vi "rtout_getTriggerConfig.vi"(0 "connection ID":refnum<k5>, 1 "axis":i32, 5 "error":errorcluster) -> (12 "polarity":i32, 14 "connection ID out":refnum<k5>, 15 "axis_out":i32, 16 "higher":i32, 17 "lower":i32, 18 "epsilon":i32, 19 "error out":errorcluster)   [LabVIEW 2016, in "amc_api.lvlib"]
doc: "Get the real time output trigger config"
uses:
  amc_api.lvlib
panel:
  out "jsonRespIn":string
  out "JSON-response":string="{\"jsonrpc\":\"2.0\",\"method\":\"\",\"params\":[5,1.245,true,\"name\"],\"id\":\"1\"}"
  out "JSON request":string
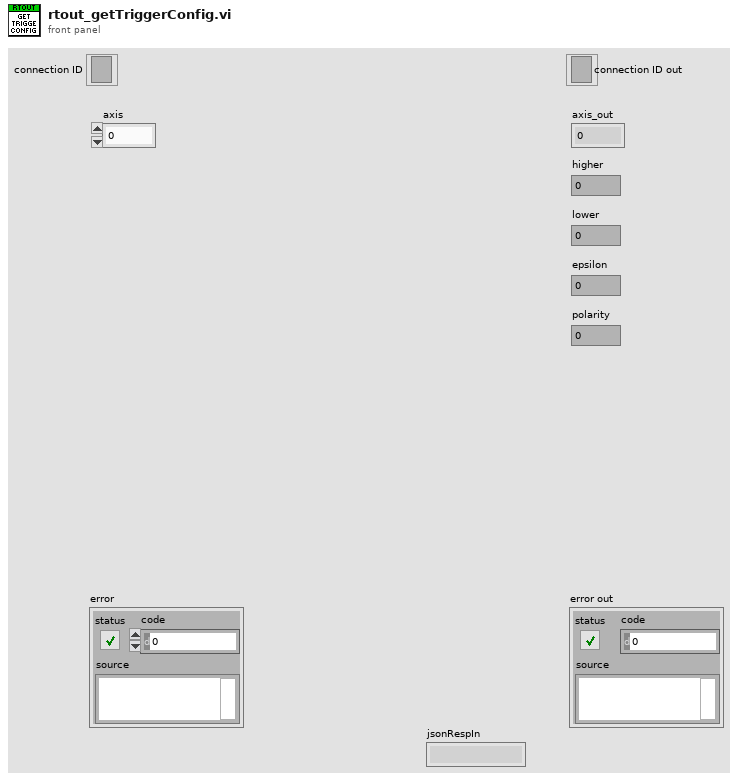
[diagram p1: front panel]
types:
  T1 = cluster{"jsonrpc":string, "method":string, "params":string[], "id":string, "api":i32, "pid":string}
  T2 = enum16{"Standard", "Buffered", "CRLF", "Immediate"}
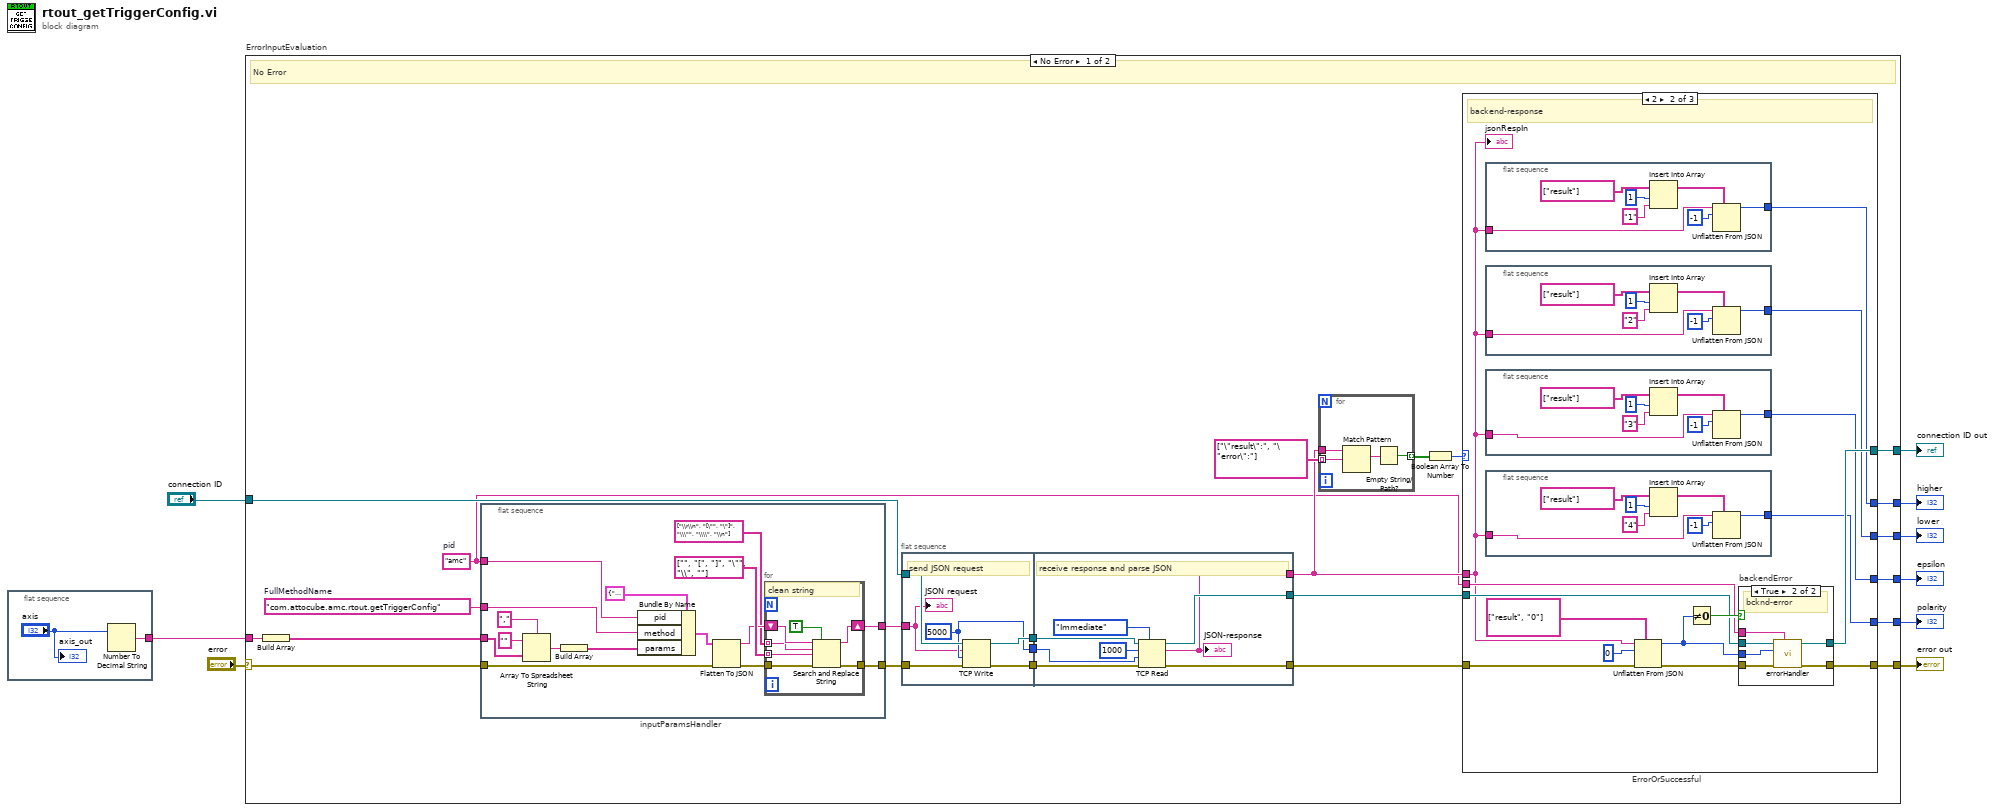
[diagram p0: block diagram]
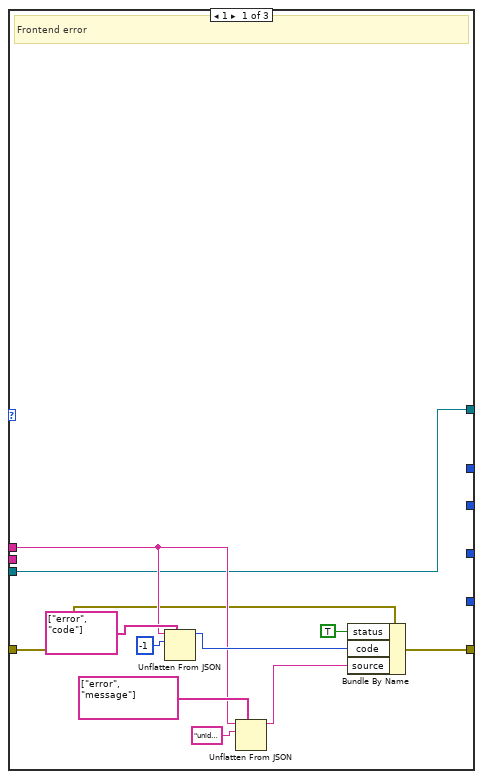
[diagram p2: hidden frame]
diagram:
  n1 = flat-sequence "in_axis" {
    tunnel: [w11] -> w5
    frame #0 {
      n2 = Number To Decimal String(number="axis") -> (decimal integer string=w11:string)  [unwired: 1 in]
      "axis_out" <- "axis"
    }
  }
  n3 = case "ErrorInputEvaluation" shown="No Error" "error" {
    selector: "error" -> [w27 w140]
    tunnel: "connection ID" -> [w31 w141]
    tunnel: [w18 w140] -> w8
    tunnel: [w19 w141] -> w7
    tunnel: w5 -> [w16 _]
    tunnel: [w15 _] -> w4
    tunnel: [w14 _] -> w3
    tunnel: [w13 _] -> w2
    tunnel: [w12 _] -> w1
    frame No Error {
      w17 = "amc"  # pid
      w28 = "com.attocube.amc.rtout.getTriggerConfig"  # FullMethodName
      # "No Error"
      n4 = Build Array ("ParametersArrayString")(w16) -> (w26:string[])
      n5 = flat-sequence "inputParamsHandler" {
        tunnel: [w104] -> w25
        tunnel: w26 -> [w110]
        tunnel: w27 -> [w109]
        tunnel: [w106] -> w24
        tunnel: w28 -> [w100]
        tunnel: w17 -> [w99]
        frame #0 {
          n6 = Array To Spreadsheet String(delimiter (Tab)=",", array=w110, 3:"" ("format string")) -> (spreadsheet string=w112:string)
          n7 = Build Array "Build Array"(w112) -> (w101:string[])
          n8 = Bundle By Name(cluster=T1 {"jsonrpc"="2.0", "method"="com.attocube.amc.res.setRESReadOutFreq", "params"=[], "id"="1", "api"=2, "pid"=""} ("Cluster"), "pid"=w99, "method"=w100, "params"=w101) -> (w111:T1)
          n9 = Flatten To JSON(anything=w111, error in (no error)=w109) -> (JSON string=w105:string, 11:w107:errorcluster)  [unwired: 1 in]
          n10 = for {
            tunnel: string[] ["\\r\\n", "[\"", "\"]", "\\\"", "\\\\", "\\n"] ("search string") -> [w118] mode=indexing
            tunnel: string[] ["", "[", "]", "\"", "\\", ""] ("replace string (\"\")") -> [w117] mode=indexing
            shift-right: [w120] -> w104
            shift-left: w105 -> [w119]
            tunnel: w107 -> [w116]
            tunnel: [w115] -> w106
            # "clean string"
            n11 = Search and Replace String(replace all?=TRUE ("replace all? (F)"), input string=w119, search string=w118, replace string=w117, error in=w116) -> (result string=w120:string, error out=w115:errorcluster)  [unwired: 3 in, 2 out]
          }
        }
      }
      n12 = flat-sequence {
        tunnel: w31 -> [w131]
        tunnel: [w129] -> w34
        tunnel: [w130] -> w33
        tunnel: w24 -> [w126]
        tunnel: [w128] -> w32
        tunnel: w25 -> [w127]
        tunnel: [w135] -> w23
        tunnel: w34 -> [w137]
        tunnel: w33 -> [w136]
        tunnel: [w133] -> w22
        tunnel: w32 -> [w134]
        tunnel: [w132] -> w21
        frame #0 {
          w128 = 5000 ("timeout ms (25000)")
          # "send JSON request"
          n13 = TCP Write(connection ID=w131, data in=w127, error in (no error)=w126, 9:w128) -> (connection ID out=w129:refnum<k5>, error out=w130:errorcluster)  [unwired: 1 out]
          "JSON request" <- w127
        }
        frame #1 {
          # "receive response and parse JSON"
          n14 = TCP Read(connection ID=w137, bytes to read=1000, error in (no error)=w136, 7:T2."Immediate" ("mode (standard)"), 9:w134) -> (connection ID out=w135:refnum<k5>, data out=w132:string, error out=w133:errorcluster)
          "JSON-response" <- w132
        }
      }
      n15 = for {
        tunnel: string[] ["\"result\":", "\"error\":"] ("path") -> [w124] mode=indexing
        tunnel: [w122] -> w29 mode=indexing
        tunnel: w21 -> [w125]
        n16 = Match Pattern(string=w125, regular expression=w124) -> (match substring=w123:string)  [unwired: 1 in, 3 out]
        n17 = Empty String/Path?(string/path=w123) -> (empty?=w122:bool)
      }
      n18 = Boolean Array To Number(Boolean array=w29) -> (number=w20:u32)
      n19 = case "ErrorOrSuccessful" shown="2" w20 {
        tunnel: w21 -> [w37 w52 _]
        tunnel: w23 -> [w35 w54 w98]
        tunnel: [w35 w53 w98] -> w19
        tunnel: [w38 w50 w97] -> w18
        tunnel: w22 -> [w36 w51 w97]
        tunnel: w17 -> [_ w55 _]
        tunnel: [_ w49 _] -> w15
        tunnel: [_ w48 _] -> w14
        tunnel: [_ w47 _] -> w13
        tunnel: [_ w46 _] -> w12
        frame 1 {
          # "Frontend error"
          n20 = Unflatten From JSON(path=string[] ["error", "code"], JSON string=w37, type and defaults=-1) -> (value=w44:i32)  [unwired: 4 in, 1 out]
          n21 = Unflatten From JSON(path=string[] ["error", "message"], JSON string=w37, type and defaults="unidentified error") -> (value=w45:string)  [unwired: 4 in, 1 out]
          n22 = Bundle By Name(cluster=w36, "status"=TRUE, "code"=w44, "source"=w45) -> (w38:errorcluster)
        }
        frame 2 {
          # "backend-response"
          n23 = flat-sequence "out_integer" {
            tunnel: w52 -> [w84]
            tunnel: [w82] -> w49
            frame #0 {
              n24 = Insert Into Array(array=string[] ["result"] ("path"), index=1, new element="1" ("idx")) -> (w86:string[])
              n25 = Unflatten From JSON(path=w86, JSON string=w84, type and defaults=-1 ("index")) -> (value=w82:i32)  [unwired: 4 in, 1 out]
            }
          }
          n26 = flat-sequence "out_integer" {
            tunnel: w52 -> [w77]
            tunnel: [w75] -> w48
            frame #0 {
              n27 = Insert Into Array(array=string[] ["result"] ("path"), index=1, new element="2" ("idx")) -> (w79:string[])
              n28 = Unflatten From JSON(path=w79, JSON string=w77, type and defaults=-1 ("index")) -> (value=w75:i32)  [unwired: 4 in, 1 out]
            }
          }
          n29 = flat-sequence "out_integer" {
            tunnel: w52 -> [w70]
            tunnel: [w68] -> w47
            frame #0 {
              n30 = Insert Into Array(array=string[] ["result"] ("path"), index=1, new element="3" ("idx")) -> (w72:string[])
              n31 = Unflatten From JSON(path=w72, JSON string=w70, type and defaults=-1 ("index")) -> (value=w68:i32)  [unwired: 4 in, 1 out]
            }
          }
          n32 = flat-sequence "out_integer" {
            tunnel: w52 -> [w63]
            tunnel: [w61] -> w46
            frame #0 {
              n33 = Insert Into Array(array=string[] ["result"] ("path"), index=1, new element="4" ("idx")) -> (w65:string[])
              n34 = Unflatten From JSON(path=w65, JSON string=w63, type and defaults=-1 ("index")) -> (value=w61:i32)  [unwired: 4 in, 1 out]
            }
          }
          n35 = Unflatten From JSON(path=string[] ["result", "0"], JSON string=w52, type and defaults=0, error in (no error)=w51) -> (value=w56:i32, error out=w58:errorcluster)  [unwired: 3 in]
          n36 = Not Equal To 0?(x=w56) -> (x != 0?=w57:bool)
          n37 = case "backendError" shown="True" w57 {
            tunnel: w56 -> [_ w96]
            tunnel: w58 -> [w90 w95]
            tunnel: [w89 w94] -> w53
            tunnel: [w90 w93] -> w50
            tunnel: w54 -> [w89 w92]
            tunnel: w55 -> [_ w91]
            frame False {
              # "successful"
            }
            frame True {
              # "bcknd-error"
              n38 = call "errorHandler.vi"("pid"=w91, "error in"=w95, "errNbr"=w96, "connection ID"=w92) -> ("error out 2"=w93:errorcluster, "connection ID out"=w94:refnum<k5>)  [unwired: 6 in]
            }
          }
          "jsonRespIn" <- w52
        }
        frame Default {
          # "NoResponse"
        }
      }
    }
    frame Error {
      # "Error"
    }
  }
  "error out" <- w8
  "connection ID out" <- w7
  "higher" <- w4
  "lower" <- w3
  "epsilon" <- w2
  "polarity" <- w1
